vi "Cannon Speed Control.vi"(1 "Cannon Global Data In":T1) -> (0 "Cannon Global Data Out":T1)   [LabVIEW 2012]
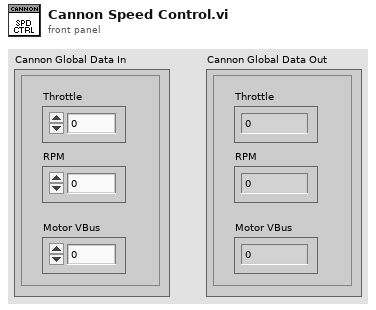
[diagram p1: front panel]
types:
  T1 = cluster{"Throttle":dbl, "RPM":dbl, "Motor VBus":dbl}
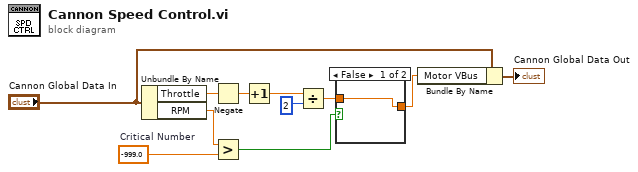
[diagram p0: block diagram]
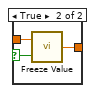
[diagram p2: hidden frame]
diagram:
  w7 = -999.0  # Critical Number
  n1 = Unbundle By Name("Cannon Global Data In") -> ("Throttle"=w3:dbl, "RPM"=w8:dbl)
  n2 = Negate(x=w3) -> (-x=w4:dbl)
  n3 = Greater?(x=w8, y=w7) -> (0:w9:bool)
  n4 = Increment(x=w4) -> (x+1=w5:dbl)
  n5 = Divide(x=w5, y=2) -> (x/y=w2:dbl)
  n6 = case shown="False" w9 {
    selector: w9 -> [_ w15]
    tunnel: w2 -> [w12 w14]
    tunnel: [w12 w13] -> w1
    frame False {
    }
    frame True {
      n7 = call "Freeze Value.vi"("Freeze Value"=w15, "In Value"=w14) -> ("Value Out"=w13:dbl)
    }
  }
  n8 = Bundle By Name(cluster="Cannon Global Data In", "Motor VBus"=w1) -> (→"Cannon Global Data Out":T1)
